vi "App_Type_FGV.vi"(8 "error in":errorcluster, 10 "Function":enum16{"Get", "Set"}(ring)) -> (0 "error out":errorcluster, 2 "App. Type":T1(ring))   [LabVIEW 2018]
panel:
  # "Inputs"
  # "Outputs"
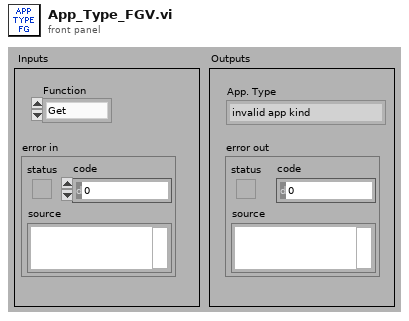
[diagram p1: front panel]
types:
  T1 = enum32{"invalid app kind", "Development System", "Run Time System", "Student Edition", "Embedded LabVIEW", "Evaluation", "Custom"}
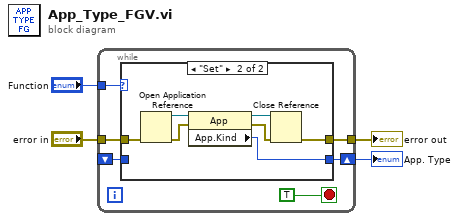
[diagram p0: block diagram]
diagram:
  n1 = while {
    tunnel: "error in" -> [w9]
    tunnel: [w8] -> w2
    tunnel: "Function" -> [w7]
    shift-right: [w10] -> w4
    shift-left: _ -> [w5]
    stop <- TRUE stop-if-true
    n2 = case shown="\"Set\"" w7 {
      tunnel: [w11 w19] -> w10
      tunnel: w9 -> [w12 w18]
      tunnel: [w12 w17] -> w8
      tunnel: w5 -> [w11 _]
      frame "Get", Default {
      }
      frame "Set" {
        n3 = Open Application Reference(8:w18) -> (0:w15:errorcluster, 3:w13:refnum<vi>)  [unwired: 3 in]
        n4 = property class="App"(reference=w13, error in=w15) -> (reference out=w14:refnum<vi>, error out=w16:errorcluster, "App.Kind"=w19:T1)
        n5 = Close Reference(reference=w14, error in (no error)=w16) -> (error out=w17:errorcluster)
      }
    }
  }
  "App. Type" <- w4
  "error out" <- w2
